vi "Bound Percent.vi"(8 "Tolerance %":dbl, 11 "Nominal":dbl) -> (0 "Min":dbl, 3 "Max":dbl)   [LabVIEW 2019]
doc: "This VI simply caculates Tolerance limits based on the \"Nominal\" value and the \"Tolerance %\""
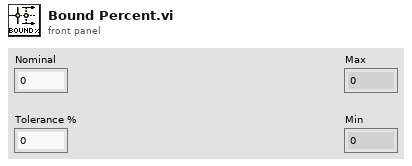
[diagram p1: front panel]
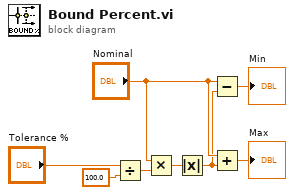
[diagram p0: block diagram]
diagram:
  n1 = Divide(x="Tolerance %", y=100.0) -> (x/y=w7:dbl)
  n2 = Multiply(x="Nominal", y=w7) -> (x*y=w5:dbl)
  n3 = Absolute Value(x=w5) -> (abs(x)=w2:dbl)
  n4 = Subtract(x="Nominal", y=w2) -> (x-y=→"Min":dbl)
  n5 = Add(x="Nominal", y=w2) -> (x+y=→"Max":dbl)
